vi "Teleop.vi"(10 "Match Info":T1={"Autonomous Elapsed Seconds"=0.0, "TeleOp Elapsed Seconds"=0.0, "Disabled Elapsed Seconds"=0.0, "Visited Autonomous"=FALSE, "Visited TeleOp"=FALSE, "Visited Disabled"=FALSE, "Autonomous Settings"={"Autonomous Style"=enum."Independent", "VI Refnum"=refnum}}, 11 "Call Context":T2) -> ()   [LabVIEW 2011]
doc: "This VI is called for each TeleOp packet received from the DS where the robot is not disabled. It is often used to read from the joysticks and update I/O or to update setpoints for timed control loops. It should complete and return within 20 milliseconds or it may miss DS packets."
uses:
  <vilib>/Rock Robotics/WPI/DriverStation/WPI_DriverStationDerivedRobotMode.ctl
  <vilib>/Rock Robotics/WPI/DriverStation/WPI_DriverStationMatch Info.ctl
  Robot Global Data.vi
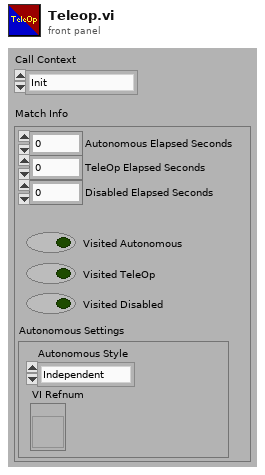
[diagram p1: front panel]
types:
  T1 = typedef "WPI_DriverStationMatch Info.ctl" = cluster{"Autonomous Elapsed Seconds":dbl, "TeleOp Elapsed Seconds":dbl, "Disabled Elapsed Seconds":dbl, "Visited Autonomous":bool, "Visited TeleOp":bool, "Visited Disabled":bool, "Autonomous Settings":cluster{"Autonomous Style":enum16{"Iterative", "Independent"}, "VI Refnum":refnum<vi>}}
  T2 = typedef "WPI_DriverStationDerivedRobotMode.ctl" = enum16{"Init", "Execute", "Stop"}
  T3 = typedef "WPI_RobotDriveDevRef.ctl" = cluster{"DevStatus":errorcluster, "Motors[]":T4[], "Square Inputs":bool, "Max Output":dbl, "Isochronous":bool}
  T4 = typedef "WPI_MotorControlDeviceRef.ctl" = cluster{"DeviceStatus":errorcluster, "Type":enum16{"PWM", "CAN"}, "PWM":cluster{"Digital Module":T5, "PWM Channel":T6, "DeadBand":T7}, "CAN":cluster{"Device Number":u8, "Control Mode":T8, "Semaphore":T9, "Max Vout":dbl}, "Invert":bool, "TransformRef":T10, "InvTransformRef":T10}
  T5 = typedef "FPGA_TypedefDigitalModule.ctl" = enum16{"Digital Module 1", "Digital Module 2"}
  T6 = typedef "FPGA_DIOPWMChannel.ctl" = enum8{"PWM 1", "PWM 2", "PWM 3", "PWM 4", "PWM 5", "PWM 6", "PWM 7", "PWM 8", "PWM 9", "PWM 10", "Invalid"}
  T7 = typedef "WPI_PWMDeadband.ctl" = cluster{"Name":string, "maxPositivePwm":i32, "minPositivePwm":i32, "centerPwm":i32, "maxNegativePwm":i32, "minNegativePwm":i32, "angularRange":u16}
  T8 = typedef "WPI_CANJaguar_ControlMode.ctl" = enum8{"Percent VBus", "Current", "Speed", "Position", "Voltage"}
  T9 = typedef "Semaphore RefNum" = refnum<k1>
  T10 = typedef "WPI_PWMTransform_ConPane.ctl" = refnum<vi>
  T11 = typedef "WPI_JoystickDevRef.ctl" = cluster{"Device":T12}
  T12 = typedef "WPI_JoystickDeviceEnum.ctl" = enum16{"USB 1", "USB 2", "USB 3", "USB 4", "Kinect 1", "Kinect 2"}
  T13 = cluster{"axis 1 (x)":i8, "axis 2 (y)":i8, "axis 3 (throttle)":i8, "axis 4":i8, "axis 5":i8, "axis 6":i8}
  T14 = typedef "WPI_JoystickButtonState.ctl" = cluster{"Button 1":bool, "Button 2":bool, "Button 3":bool, "Button 4":bool, "Button 5":bool, "Button 6":bool, "Button 7":bool, "Button 8":bool, "Button 9":bool, "Button 10":bool, "Button 11":bool, "Button 12":bool}
  T15 = typedef "FPGA_WatchdogDevRef.ctl" = cluster{"DevStatus":errorcluster}
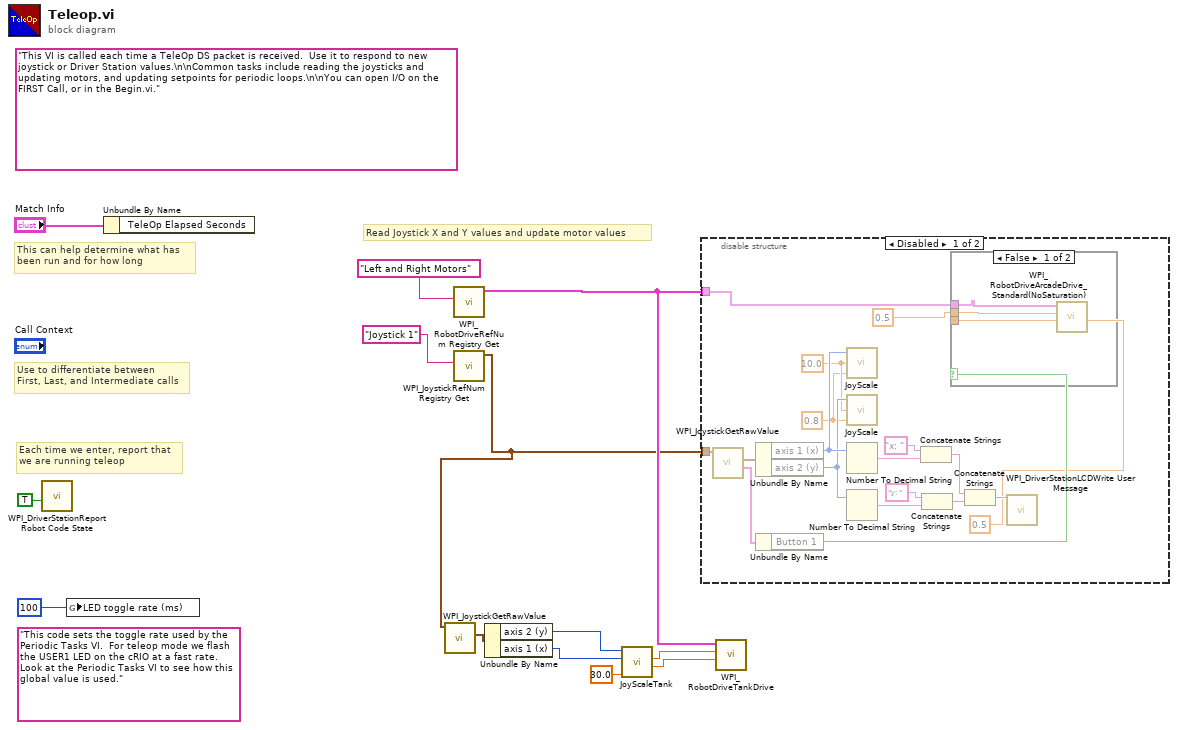
[diagram p0: block diagram]
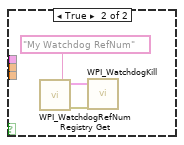
[diagram p2: hidden frame]
diagram:
  (unwired) "This code sets the toggle rate used by the Periodic Tasks VI.  For teleop mode we flash the USER1 LED on the cRIO at a fast rate.  Look at the Periodic Tasks VI to see how this global value is used."
  (unwired) "This VI is called each time a TeleOp DS packet is received.  Use it to respond to new joystick or Driver Station values.\n\nCommon tasks include reading the joysticks and updating motors, and updating setpoints for periodic loops.\n\nYou can open I/O on the FIRST Call, or in the Begin.vi."
  # "Each time we enter, report that\nwe are running teleop"
  # "Use to differentiate between\nFirst, Last, and Intermediate calls"
  # "This can help determine what has\nbeen run and for how long"
  # "Read Joystick X and Y values and update motor values"
  n1 = call <vilib>:"WPI_DriverStationReport Robot Code State.vi"("TeleOp"=TRUE ("Autonomous")) -> ()  [unwired: 10 in, 1 out]
  n2 = global write "Robot Global Data.vi" "LED toggle rate (ms)"(u32 100 ("LED ms toggle rate")) -> ()
  n3 = Unbundle By Name("Match Info") -> ()  [unwired: 1 out]
  n4 = call <vilib>:"WPI_RobotDriveRefNum Registry Get.vi"("refnum name"="Left and Right Motors") -> ("RobotDriveDevRef"=w2:T3)  [unwired: 1 in, 9 out]
  n5 = call <vilib>:"WPI_JoystickRefNum Registry Get.vi"("refnum name"="Joystick 1") -> ("JoystickDevRef"=w1:T11)  [unwired: 1 in, 9 out]
  n6 = call <vilib>:"WPI_JoystickGetRawValue.vi"("JoystickDevRef"=w1) -> ("Axes"=w8:T13)  [unwired: 8 in, 2 out]
  n7 = Unbundle By Name(w8) -> ("axis 2 (y)"=w7:i8, "axis 1 (x)"=w6:i8)
  n8 = call "JoyScaleTank.vi"("Tolerance"=30.0, "x Axis"=w6, "y Axis"=w7) -> ("Speed Right"=w3:dbl, "Speed Left"=w4:dbl)  [unwired: 6 in, 1 out]
  n9 = disable-structure shown="Disabled" {
    disable-tunnel: w1 -> [w26 _]
    disable-tunnel: w2 -> [w25 _]
    frame Disabled {
      w17 = 0.8 ("Max Power")
      w18 = 10.0 ("DeadZone")
      n10 = call <vilib>:"WPI_JoystickGetRawValue.vi"("JoystickDevRef"=w26) -> ("Buttons"=w28:T14, "Axes"=w31:T13)  [unwired: 8 in, 1 out]
      n11 = Unbundle By Name(w31) -> ("axis 1 (x)"=w30:i8, "axis 2 (y)"=w29:i8)
      n12 = Unbundle By Name(w28) -> ("Button 1"=w27:bool)
      n13 = call "JoyScale.vi"("Max Power"=w17, "DeadZone"=w18, "JoyValue"=w30) -> ()  [unwired: 1 out]
      n14 = call "JoyScale.vi"("Max Power"=w17, "DeadZone"=w18, "JoyValue"=w29) -> ()  [unwired: 1 out]
      n15 = Number To Decimal String(number=w30) -> (decimal integer string=w23:string)  [unwired: 1 in]
      n16 = Number To Decimal String(number=w29) -> (decimal integer string=w21:string)  [unwired: 1 in]
      n17 = Concatenate Strings("x: " ("string"), w23) -> (w20:string)
      n18 = Concatenate Strings("y: " ("string"), w21) -> (w19:string)
      n19 = case shown="False" w27 {
        tunnel: w25 -> [w34 _]
        tunnel: 0.5 -> [w33 _]
        tunnel: 0.5 -> [w32 _]
        frame False {
          n20 = call <vilib>:"WPI_RobotDriveArcadeDrive_Standard(NoSaturation).vi"("Y axis value"=w32, "X axis value"=w33, "RobotDriveDevRef"=w34) -> ()  [unwired: 1 in, 8 out]
        }
        frame True {
          n21 = call <vilib>:"WPI_WatchdogRefNum Registry Get.vi"("refnum name"="My Watchdog RefNum") -> ("error out"=w37:errorcluster, "WatchdogDevRef"=w36:T15)  [unwired: 9 in]
          n22 = call <vilib>:"WPI_WatchdogKill.vi"("error in (no error)"=w37, "WatchdogDevRef"=w36) -> ()  [unwired: 8 in, 2 out]
        }
      }
      n23 = Concatenate Strings(w20, w19) -> (w16:string)
      n24 = call <vilib>:"WPI_DriverStationLCDWrite User Message.vi"("line text"=w16) -> ()  [unwired: 14 in, 1 out]
    }
    frame Enabled {
    }
  }
  n25 = call <vilib>:"WPI_RobotDriveTankDrive.vi"("Right axis value"=w3, "Left axis value"=w4, "RobotDriveDevRef"=w2) -> ()  [unwired: 7 in, 2 out]
